vi "getJobOpeningsAmount.vi"(8 "errorIn":errorcluster, 11 "staisticsData":T1) -> (0 "errorOut":errorcluster, 3 "statistics":cluster{cluster{"X":dbl, "Y":dbl}[]}[](array[cluster]))   [LabVIEW 2025]
uses:
  control/statisticsData.ctl
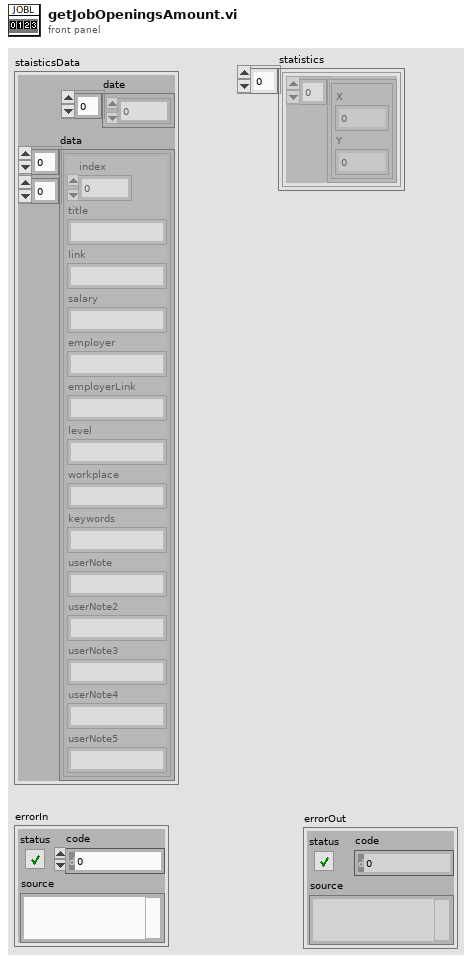
[diagram p1: front panel]
types:
  T1 = typedef "statisticsData.ctl" = cluster{"date":dbl[], "data":cluster{"index":i32, "title":string, "link":string, "salary":string, "employer":string, "employerLink":string, "level":string, "workplace":string, "keywords":string, "userNote":string, "userNote2":string, "userNote3":string, "userNote4":string, "userNote5":string}[][]}
  T2 = cluster{"index":i32, "title":string, "link":string, "salary":string, "employer":string, "employerLink":string, "level":string, "workplace":string, "keywords":string, "userNote":string, "userNote2":string, "userNote3":string, "userNote4":string, "userNote5":string}[][]
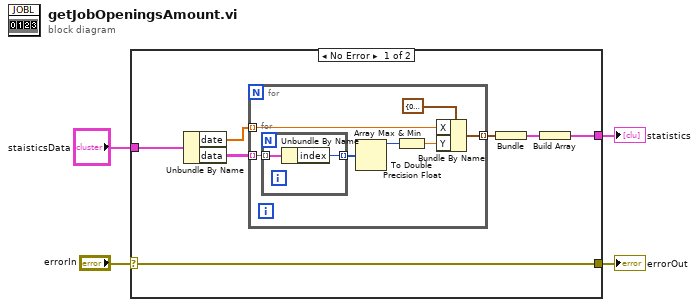
[diagram p0: block diagram]
diagram:
  n1 = case shown="No Error" "errorIn" {
    selector: "errorIn" -> [w5 w21]
    tunnel: [w11 _] -> w4
    tunnel: "staisticsData" -> [w6 _]
    tunnel: [w5 w21] -> w1
    frame No Error {
      n2 = Unbundle By Name(w6) -> ("date"=w7:dbl[], "data"=w8:T2)
      n3 = for {
        tunnel: w7 -> [w16] mode=indexing
        tunnel: w8 -> [w15] mode=indexing
        tunnel: [w12] -> w9 mode=indexing
        n4 = for {
          tunnel: w15 -> [w20] mode=indexing
          tunnel: [w19] -> w14 mode=indexing
          n5 = Unbundle By Name(w20) -> ("index"=w19:i32)
        }
        n6 = Array Max & Min(array=w14) -> (max value=w13:i32)  [unwired: 3 out]
        n7 = To Double Precision Float(number=w13) -> (double precision float=w18:dbl)
        n8 = Bundle By Name(cluster=cluster{"X":dbl, "Y":dbl} {"X"=0.0, "Y"=0.0}, "X"=w16, "Y"=w18) -> (w12:cluster{"X":dbl, "Y":dbl})
      }
      n9 = Bundle(w9) -> (w10:cluster{cluster{"X":dbl, "Y":dbl}[]})  [unwired: 1 in]
      n10 = Build Array(w10) -> (w11:cluster{cluster{"X":dbl, "Y":dbl}[]}[])
    }
    frame Error {
    }
  }
  "statistics" <- w4
  "errorOut" <- w1
